vi "Close Queue.vi"(8 "error in (no error)":errorcluster, 10 "Kill Now? (T)":bool=TRUE, 11 "DbMeasurement in":refnum<class "DbMeasurement.lvclass">) -> (0 "error out":errorcluster, 3 "DbMeasurement out":refnum<class "DbMeasurement.lvclass">)   [LabVIEW 2013, in "DbMeasurement.lvclass"]
doc: "This private method closes the queue used to store database values. By default, it closes the queue immediately. If an input Boolean is True, it will wait until the queue is empty or for 10 seconds, whichever comes first, and then close the queue. This VI executes normally even if an error occurs before hand."
uses:
  DbMeasurement.lvclass
  DbMeasurement.lvclass/DbMeasurement.ctl
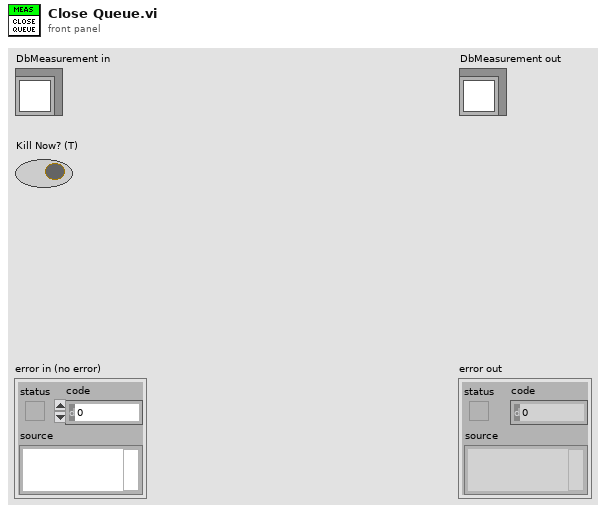
[diagram p1: front panel]
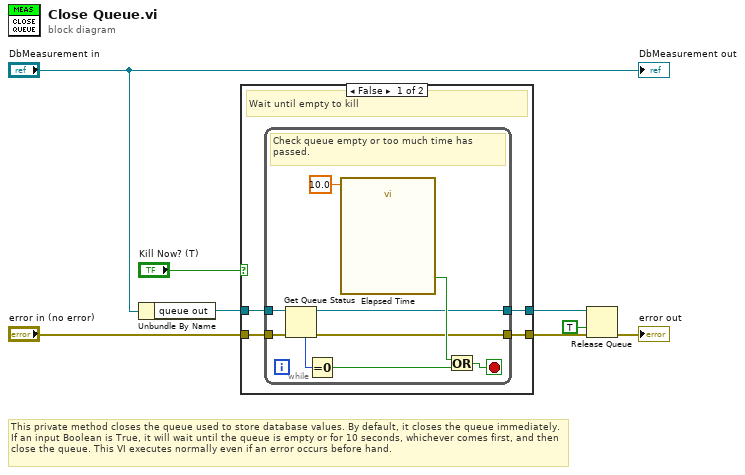
[diagram p0: block diagram]
diagram:
  # "This private method closes the queue used to store database values. By default, it closes the queue immediately. If an input Boolean is True, it will wait until the queue is empty or for 10 seconds, whichever comes first, and then close the queue. This VI executes normally even if an error occurs before hand."
  n1 = Unbundle By Name("DbMeasurement in") -> ("queue out"=w2:refnum<queue>)
  n2 = case shown="False" "Kill Now? (T)" {
    tunnel: "error in (no error)" -> [w12 w23]
    tunnel: [w11 w23] -> w3
    tunnel: w2 -> [w10 w22]
    tunnel: [w9 w22] -> w1
    frame False {
      # "Wait until empty to kill"
      n3 = while {
        tunnel: w12 -> [w21]
        tunnel: [w16] -> w11
        tunnel: w10 -> [w15]
        tunnel: [w14] -> w9
        stop <- w19 stop-if-true
        # "Check queue empty or too much time has passed."
        n4 = Get Queue Status(queue=w15, error in (no error)=w21) -> (queue out=w14:refnum<queue>, error out=w16:errorcluster, # elements in queue=w20:i32)  [unwired: 1 in, 5 out]
        n5 = Equal To 0?(x=w20) -> (x = 0?=w18:bool)
        n6 = call "Elapsed Time"("Time Target (s)"=10.0) -> ("Time has Elapsed"=w17:bool)  [unwired: 11 in, 7 out]
        n7 = Or(x=w17, y=w18) -> (x .or. y?=w19:bool)
      }
    }
    frame True {
      # "Kill queue immediately"
    }
  }
  n8 = Release Queue(queue=w1, force destroy? (F)=TRUE, error in (no error)=w3) -> (error out=→"error out":errorcluster)  [unwired: 2 out]
  "DbMeasurement out" <- "DbMeasurement in"
